vi "main.vi"() -> ()   [LabVIEW 2018]
uses:
  Program Files (x86)/National Instruments/LabVIEW 2018/examples/Connectivity/Python/support/PythonVersionsEnum.ctl
  <vilib>/LabVIEW Interface for Arduino/LabVIEW Interface for Arduino.lvlib
panel:
  in  "dy offset":dbl=2.0
  out "X 2":i32=372
  out "Y 2":i32=259
  out "dx":dbl=3.0
  out "dy":dbl=-1.0
  in  "wait":u32=5
  out "element 2":string
  out "element":string
  out "x .or. y?":bool
  out "output variable 2":dbl=116.25
  out "output variable":dbl=79.28571428571428
  in  "Ydown":i16=120
  in  "Yup":i16=150
  in  "Xdown":i16=35
  in  "Xup":i16=75
  out "Y":i32=267
  out "X":i32=291
  in  "VISA resource":refnum<visa-resource-name>="COM8"
  out "error out 2":errorcluster={"status"=TRUE, "code"=1672, "source"="Python Node in test3_2.vi<APPEND>\n\nModule Path: C:\\Users\\2251338l\\OD\\Member\\Asfand\\GazeTracking\\test3_2.py\nFunction Name: get"}
  in  "stop":bool
  out "error out":errorcluster={"status"=TRUE, "code"=1672, "source"="Python Node in test3_2.vi<APPEND>\n\nModule Path: C:\\Users\\2251338l\\OD\\Member\\Asfand\\GazeTracking\\test3_2.py\nFunction Name: get"}
  # "Gaze tracking machine"
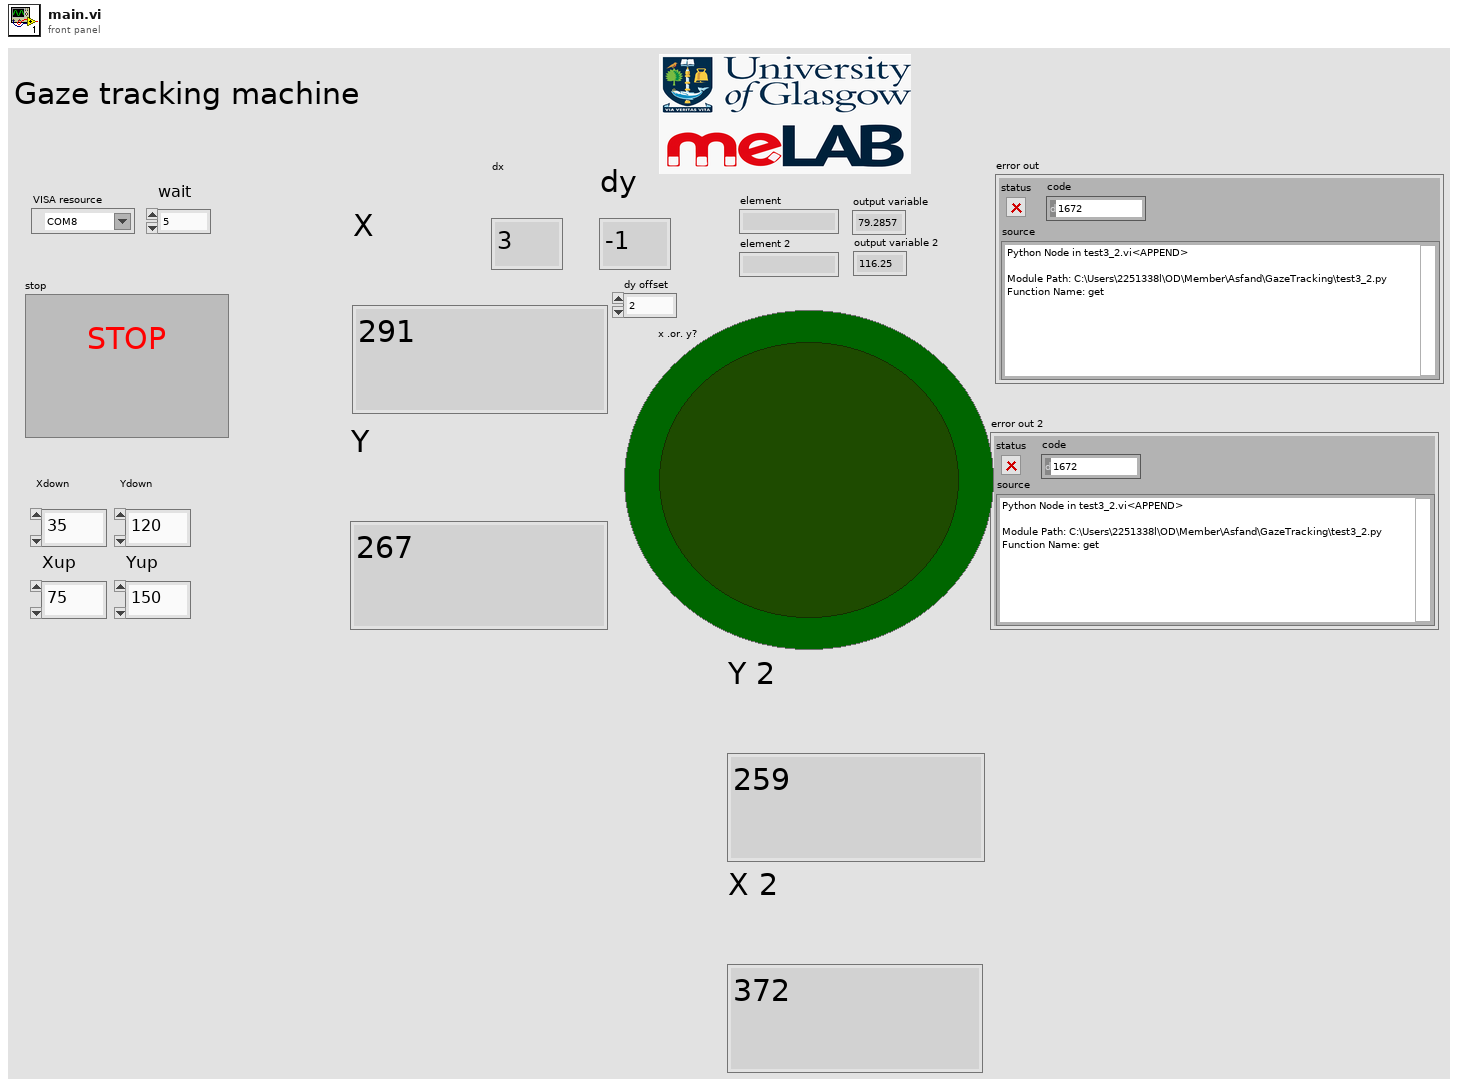
[diagram p1: front panel]
types:
  T1 = typedef "PythonVersionsEnum.ctl" = enum16{"2.7", "3.6"}
  T2 = typedef "LabVIEW Interface for Arduino.lvlib/Arduino Resource.ctl" = cluster{"VISA resource":refnum<visa-resource-name>, "Board Type":T3, "Connection Type":enum8{"USB / Serial"}, "Bytes Per Packet (15)":u8}
  T3 = typedef "LabVIEW Interface for Arduino.lvlib/Board Type.ctl" = enum16{"Uno", "Dimuelanove w/Atmega 328", "Mega 2560"}
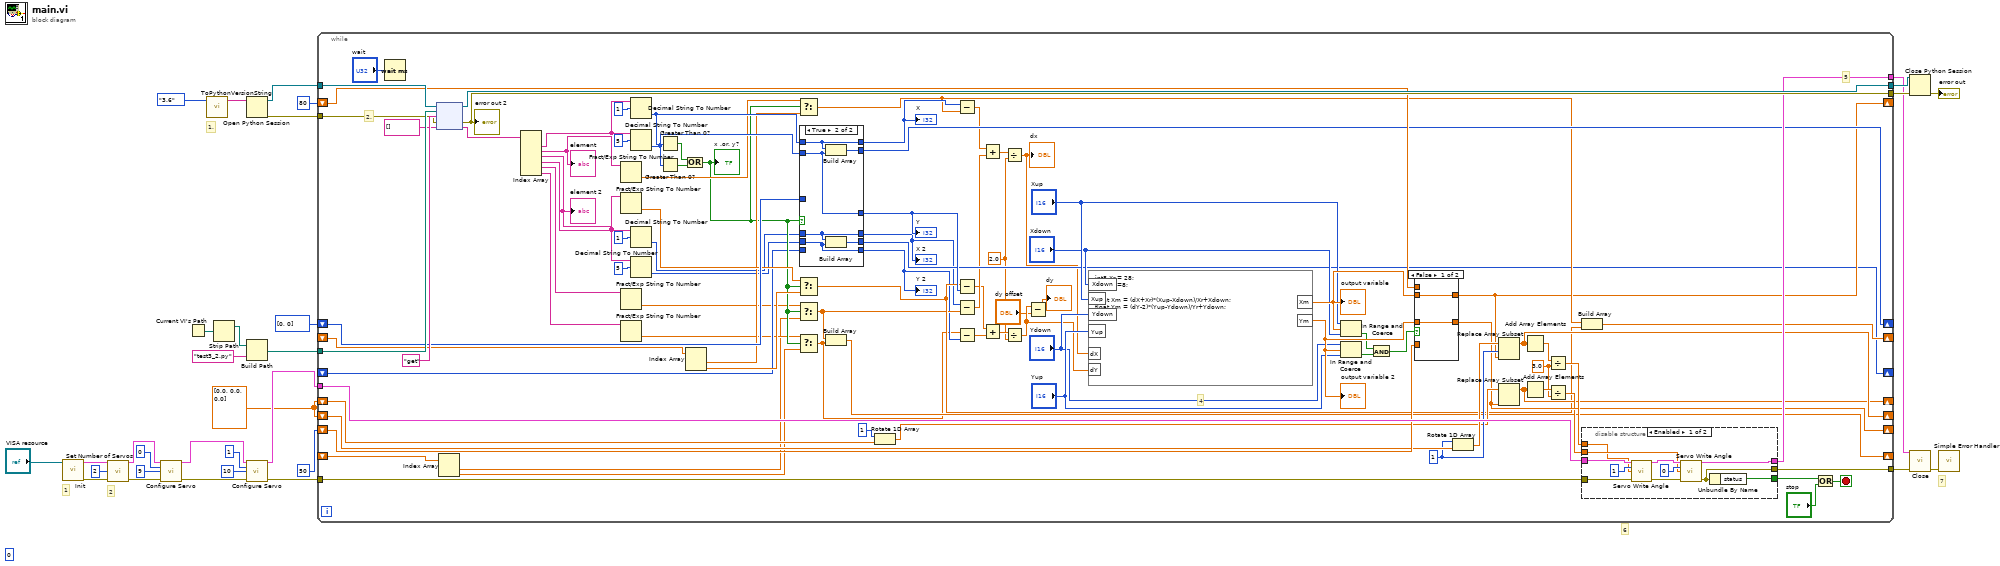
[diagram p0: block diagram]
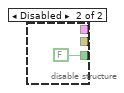
[diagram p2: hidden frame]
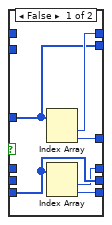
[diagram p3: hidden frame]
diagram:
  w1 = dbl[] [0.0, 0.0, 0.0]
  (unwired) 0 ("offset")
  # "7"
  # "6"
  # "2"
  # "1"
  # "1."
  n1 = call <vilib>:"Init.vi"("VISA resource"="VISA resource") -> ("Arduino Resource"=w21:T2, "error out"=w20:errorcluster)  [unwired: 17 in]
  n2 = call <vilib>:"Set Number of Servos.vi"("Arduino Resource"=w21, "Number Of Servos (1)"=u8 2 ("Number of Servos"), "error in"=w20) -> ("Arduino Resource"=w19:T2, "error out"=w18:errorcluster)  [unwired: 11 in]
  n3 = call <vilib>:"Configure Servo.vi"("Arduino Resource"=w19, "Servo Number (0)"=u8 0 ("Servo Number"), "DIO Pin (2)"=u8 9 ("Servo Number"), "error in"=w18) -> ("Arduino Resource"=w17:T2, "error out"=w16:errorcluster)  [unwired: 10 in]
  n4 = Current VI's Path() -> (path=w30:path)
  n5 = call "ToPythonVersionString.vi"("python version"=PythonVersionsEnum."3.6") -> ("python version string"=w24:string)  [unwired: 10 in]
  n6 = Strip Path(path=w30) -> (stripped path=w29:path)  [unwired: 1 out]
  n7 = Open Python Session(python version=w24) -> (session out=w23:refnum<k35>, error out=w22:errorcluster)  [unwired: 2 in]
  n8 = Build Path(base path=w29, name or relative path="test3_2.py") -> (appended path=w27:path)
  n9 = call <vilib>:"Configure Servo.vi"("Arduino Resource"=w17, "Servo Number (0)"=u8 1 ("Servo Number"), "DIO Pin (2)"=u8 10 ("Servo Number"), "error in"=w16) -> ("Arduino Resource"=w9:T2, "error out"=w8:errorcluster)  [unwired: 10 in]
  n10 = while {
    tunnel: w27 -> [w126]
    tunnel: [w124] -> w26
    tunnel: [w123] -> w25
    tunnel: w23 -> [w122]
    tunnel: w22 -> [w121]
    tunnel: w9 -> [w119]
    tunnel: w8 -> [w118]
    tunnel: [w117] -> w6
    tunnel: [w116] -> w5
    shift-right: [w76] -> _
    shift-left: i16 80 -> [w110]
    shift-right: [w69] -> _
    shift-left: i16 50 -> [w109]
    shift-right: [w97] -> _
    shift-left: i32[] [0, 0] -> [w96]
    shift-right: [w84] -> _
    shift-left: _ -> [w83]
    shift-right: [w67] -> _
    shift-left: w1 -> [w78]
    shift-right: [w66] -> _
    shift-left: w1 -> [w70]
    shift-right: [w57] -> _
    shift-left: _ -> [w56]
    shift-right: [w55] -> _
    shift-left: _ -> [w51]
    stop <- w114 stop-if-true
    w36 = 2.0 ("y")
    w65 = 3.0 ("y")
    w77 = 1 ("n")
    # "4"
    # "5"
    # "2."
    n11 = Wait (ms)(milliseconds to wait="wait") -> ()  [unwired: 1 out]
    n12 = node(w122, w126, "get" ("function name"), w121, string[] []) -> (w124:refnum<k35>, w123:errorcluster, w92:string[])  [unwired: 2 out]
    "error out 2" <- w123
    n13 = Index Array(array=w51) -> (element #1=w49:dbl, element #2=w48:dbl)  [unwired: 2 in]
    n14 = Index Array(array=w92) -> (element #1=w91:string, element #2=w90:string, element #3=w89:string, element #4=w61:string, element #5=w54:string, element #6=w53:string)  [unwired: 6 in]
    "element" <- w90
    "element 2" <- w89
    n15 = Fract/Exp String To Number(string=w90) -> (number=w87:dbl)  [unwired: 3 in, 1 out]
    n16 = Fract/Exp String To Number(string=w89) -> (number=w86:dbl)  [unwired: 3 in, 1 out]
    n17 = Fract/Exp String To Number(string=w54) -> (number=w52:dbl)  [unwired: 3 in, 1 out]
    n18 = Fract/Exp String To Number(string=w53) -> (number=w50:dbl)  [unwired: 3 in, 1 out]
    n19 = Decimal String To Number(string=w91, offset=1) -> (number=w100:i32)  [unwired: 1 in, 1 out]
    n20 = Decimal String To Number(string=w91, offset=5) -> (number=w99:i32)  [unwired: 1 in, 1 out]
    n21 = Decimal String To Number(string=w61, offset=1) -> (number=w59:i32)  [unwired: 1 in, 1 out]
    n22 = Decimal String To Number(string=w61, offset=5) -> (number=w58:i32)  [unwired: 1 in, 1 out]
    n23 = Greater Than 0?(x=w100) -> (x > 0?=w102:bool)
    n24 = Greater Than 0?(x=w99) -> (x > 0?=w101:bool)
    n25 = Or(x=w102, y=w101) -> (x .or. y?=w60:bool)
    "x .or. y?" <- w60
    n26 = Index Array(array=w83) -> (element #1=w82:dbl, element #2=w81:dbl)  [unwired: 2 in]
    n27 = Select(t=w87, s=w60, f=w82) -> (s? t:f=w85:dbl)
    n28 = Select(t=w86, s=w60, f=w81) -> (s? t:f=w64:dbl)
    n29 = Select(t=w52, s=w60, f=w49) -> (s? t:f=w46:dbl)
    n30 = Select(t=w50, s=w60, f=w48) -> (s? t:f=w44:dbl)
    n31 = case shown="True" w60 {
      tunnel: w100 -> [_ w150]
      tunnel: w99 -> [_ w149]
      tunnel: [w144 w150] -> w98
      tunnel: [w143 w149] -> w80
      tunnel: [w142 w148] -> w97
      tunnel: w96 -> [w142 _]
      tunnel: w59 -> [_ w147]
      tunnel: w58 -> [_ w146]
      tunnel: [w139 w147] -> w47
      tunnel: [w140 w146] -> w45
      tunnel: [w141 w145] -> w57
      tunnel: w56 -> [w141 _]
      frame False {
        n32 = Index Array(array=w142) -> (element #1=w144:i32, element #2=w143:i32)  [unwired: 2 in]
        n33 = Index Array(array=w141) -> (element #1=w139:i32, element #2=w140:i32)  [unwired: 2 in]
      }
      frame True {
        n34 = Build Array(w150, w149) -> (w148:i32[])
        n35 = Build Array(w147, w146) -> (w145:i32[])
      }
    }
    "X" <- w98
    "Y" <- w80
    "Y 2" <- w45
    "X 2" <- w47
    n36 = Build Array(w46, w44) -> (w55:dbl[])
    n37 = Rotate 1D Array(1:w70, 2:1 ("n")) -> (0:w71:dbl[])
    n38 = Subtract(x=w98, y=w85) -> (x-y=w43:dbl)
    n39 = Subtract(x=w64, y=w80) -> (x-y=w39:dbl)
    n40 = Subtract(x=w47, y=w46) -> (x-y=w42:dbl)
    n41 = Subtract(x=w44, y=w45) -> (x-y=w38:dbl)
    n42 = Add(x=w43, y=w42) -> (x+y=w41:dbl)
    n43 = Add(x=w39, y=w38) -> (x+y=w37:dbl)
    n44 = Divide(x=w41, y=w36) -> (x/y=w40:dbl)
    "dx" <- w40
    n45 = Divide(x=w37, y=w36) -> (x/y=w35:dbl)
    n46 = Subtract(x=w35, y="dy offset") -> (x-y=→"dy":dbl)
    n47 = formula code="int8 Xr = 28;\nint8 Yr =8;\n\nfloat Xm = (dX+Xr)*(Xup-Xdown)/Xr+Xdown;\nfloat Ym = (dY-2)*(Yup-Ydown)/Yr+Ydown;"("dX"=w40, "dY"=w35, "Xdown"="Xdown", "Xup"="Xup", "Ydown"="Ydown", "Yup"="Yup") -> ("Xm"=w108:dbl, "Ym"=w105:dbl)
    "output variable" <- w108
    "output variable 2" <- w105
    n48 = In Range and Coerce(upper limit="Xup", x=w108, lower limit="Xdown") -> (In Range?=w104:bool)  [unwired: 1 out]
    n49 = In Range and Coerce(upper limit="Ydown", x=w105, lower limit="Yup") -> (In Range?=w103:bool)  [unwired: 1 out]
    n50 = And(x=w104, y=w103) -> (x .and. y?=w111:bool)
    n51 = case shown="False" w111 {
      tunnel: w108 -> [w152 w154]
      tunnel: [w152 w154] -> w76
      tunnel: w105 -> [w151 w153]
      tunnel: [w151 w153] -> w69
      tunnel: w110 -> [_ _]
      tunnel: w109 -> [_ _]
      frame False {
      }
      frame True {
      }
    }
    n52 = Rotate 1D Array(1:w78, 2:w77) -> (0:w79:dbl[])
    n53 = Replace Array Subset(array=w79, new element=w76, index=w77) -> (w67:dbl[])
    n54 = Replace Array Subset(array=w71, new element=w69) -> (w66:dbl[])  [unwired: 1 in]
    n55 = Add Array Elements(numeric array=w67) -> (sum=w75:dbl)
    n56 = Add Array Elements(numeric array=w66) -> (sum=w73:dbl)
    n57 = Divide(x=w75, y=w65) -> (x/y=w74:dbl)
    n58 = Divide(x=w73, y=w65) -> (x/y=w68:dbl)
    n59 = Build Array(w85, w64) -> (w84:dbl[])
    n60 = disable-structure shown="Enabled" {
      disable-tunnel: [w137 FALSE ("status")] -> w120
      disable-tunnel: w119 -> [w136 _]
      disable-tunnel: w118 -> [w135 _]
      disable-tunnel: [w134 _] -> w117
      disable-tunnel: [w133 _] -> w116
      disable-tunnel: w68 -> [w128 _]
      disable-tunnel: w74 -> [w127 _]
      frame Enabled {
        n61 = call <vilib>:"Servo Write Angle.vi"("Arduino Resource"=w136, "Servo Number"=u8 1, "Angle (Degrees)"=w127, "error in"=w135) -> ("Arduino Resource"=w131:T2, "error out"=w132:errorcluster)  [unwired: 10 in]
        n62 = call <vilib>:"Servo Write Angle.vi"("Arduino Resource"=w131, "Servo Number"=u8 0, "Angle (Degrees)"=w128, "error in"=w132) -> ("Arduino Resource"=w133:T2, "error out"=w134:errorcluster)  [unwired: 10 in]
        n63 = Unbundle By Name(w134) -> ("status"=w137:bool)
      }
      frame Disabled {
      }
    }
    n64 = Or(x=w120, y="stop") -> (x .or. y?=w114:bool)
  }
  n65 = Close Python Session(session in=w26, error in=w25) -> (11:→"error out":errorcluster)
  n66 = call <vilib>:"Close.vi"("Arduino Resource"=w5, "error in"=w6) -> ("error out"=w7:errorcluster)  [unwired: 13 in]
  n67 = call <vilib>:"Simple Error Handler.vi"("error in (no error)"=w7) -> ()  [unwired: 4 in, 5 out]
